vi "PtoP.vi"(3 "Spacing":dbl, 5 "LineNo":i32, 6 "Direction":enum16{"Y to X", "X to Y"}(ring), 7 "Step":dbl, 8 "error in":errorcluster, 9 "Wait time":i32, 10 "Length":i32, 11 "StartPos":dbl[](array[numeric])) -> (0 "error out":errorcluster)   [LabVIEW 2022 SP3]
uses:
  Global 3.vi
  Newport.XPS.CommandInterface
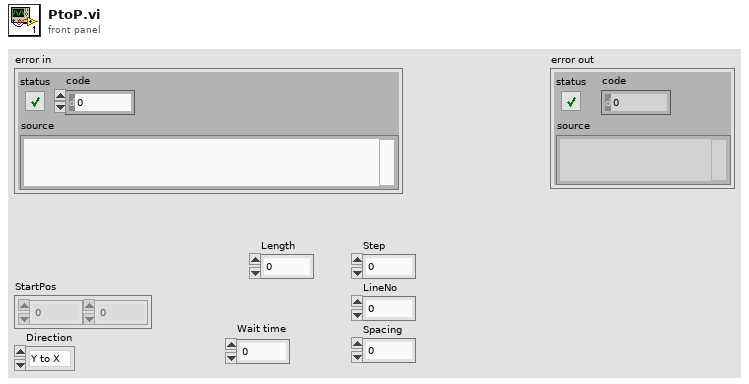
[diagram p1: front panel]
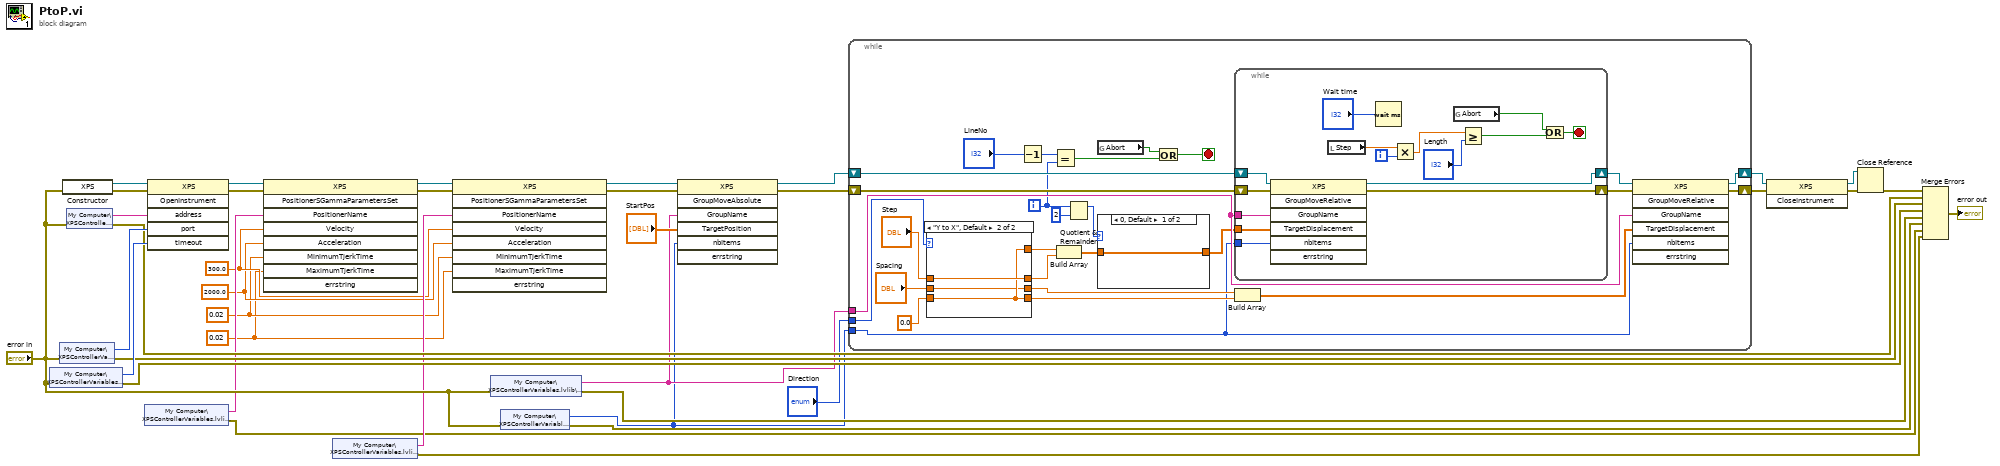
[diagram p0: block diagram]
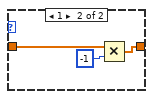
[diagram p2: hidden frame]
diagram:
  w11 = 0.02 ("MaxJT")
  w12 = 0.02 ("MinJT")
  w13 = 2000.0 ("Acc")
  w14 = 300.0 ("Vel")
  n1 = shared-variable "My Computer\\XPSControllerVariables.lvlib\\Timeout"(error in="error in") -> (w33:i16, error out=w28:errorcluster)
  n2 = shared-variable "My Computer\\XPSControllerVariables.lvlib\\Port"(error in="error in") -> (w34:i16, error out=w29:errorcluster)
  n3 = constructor class="XPS"(error in="error in") -> (reference out=w37:refnum<k24>, error out=w36:errorcluster)  [unwired: 2 in, 1 out]
  n4 = shared-variable "My Computer\\XPSControllerVariables.lvlib\\IP"(error in="error in") -> (w35:string, error out=w30:errorcluster)
  n5 = shared-variable "My Computer\\XPSControllerVariables.lvlib\\PosNameX"() -> (w16:string, error out=w9:errorcluster)  [unwired: 1 in]
  n6 = invoke class="XPS" method="OpenInstrument"(reference=w37, error in=w36, "address"=w35, "port"=w34, "timeout"=w33) -> (reference out=w22:refnum<k24>, error out=w21:errorcluster)  [unwired: 1 in, 4 out]
  n7 = invoke class="XPS" method="PositionerSGammaParametersSet"(reference=w22, error in=w21, "PositionerName"=w16, "Velocity"=w14, "Acceleration"=w13, "MinimumTjerkTime"=w12, "MaximumTjerkTime"=w11) -> (reference out=w20:refnum<k24>, error out=w19:errorcluster)  [unwired: 2 in, 7 out]
  n8 = shared-variable "My Computer\\XPSControllerVariables.lvlib\\PosNameY"() -> (w15:string, error out=w8:errorcluster)  [unwired: 1 in]
  n9 = invoke class="XPS" method="PositionerSGammaParametersSet"(reference=w20, error in=w19, "PositionerName"=w15, "Velocity"=w14, "Acceleration"=w13, "MinimumTjerkTime"=w12, "MaximumTjerkTime"=w11) -> (reference out=w18:refnum<k24>, error out=w17:errorcluster)  [unwired: 2 in, 7 out]
  n10 = shared-variable "My Computer\\XPSControllerVariables.lvlib\\GroupName"(error in="error in") -> (w3:string, error out=w27:errorcluster)
  n11 = shared-variable "My Computer\\XPSControllerVariables.lvlib\\nbitem"(error in="error in") -> (w2:i16, error out=w23:errorcluster)
  n12 = invoke class="XPS" method="GroupMoveAbsolute"(reference=w18, error in=w17, "GroupName"=w3, "TargetPosition"="StartPos", "nbItems"=w2) -> (reference out=w7:refnum<k24>, error out=w6:errorcluster)  [unwired: 2 in, 5 out]
  n13 = while {
    tunnel: w3 -> [w45]
    tunnel: w2 -> [w39]
    shift-right: [w47] -> w5
    shift-left: w7 -> [w64]
    shift-right: [w46] -> w4
    shift-left: w6 -> [w63]
    tunnel: "Direction" -> [w49]
    i -> [w44]
    stop <- w57 stop-if-true
    n14 = case shown="\"Y to X\", Default" w49 {
      tunnel: [w86 w88] -> w56
      tunnel: "Step" -> [w86 w89]
      tunnel: [w85 w89] -> w54
      tunnel: 0.0 -> [w85 w88]
      tunnel: [w85 w87] -> w52
      tunnel: [w84 w88] -> w51
      tunnel: "Spacing" -> [w84 w87]
      frame "X to Y" {
      }
      frame "Y to X", Default {
      }
    }
    n15 = Decrement(x="LineNo") -> (x-1=w60:i32)
    n16 = Equal?(x=w60, y=w44) -> (x = y?=w58:bool)
    n17 = Build Array(w56, w54) -> (w42:dbl[])
    n18 = Quotient & Remainder(x=w44, y=2) -> (x-y*floor(x/y)=w40:i32)  [unwired: 1 out]
    n19 = global read "Global 3.vi" "Abort"() -> (w59:bool)
    n20 = case shown="0, Default" w40 {
      tunnel: w42 -> [w80 w82]
      tunnel: [w80 w81] -> w41
      frame 0, Default {
      }
      frame 1 {
        n21 = Multiply(x=w82, y=-1) -> (x*y=w81:dbl[])
      }
    }
    n22 = Or(x=w59, y=w58) -> (x .or. y?=w57:bool)
    n23 = while {
      tunnel: w45 -> [w75]
      tunnel: w41 -> [w74]
      tunnel: w39 -> [w73]
      shift-right: [w77] -> w62
      shift-left: w64 -> [w79]
      shift-right: [w76] -> w61
      shift-left: w63 -> [w78]
      i -> [w71]
      stop <- w65 stop-if-true
      n24 = invoke class="XPS" method="GroupMoveRelative"(reference=w79, error in=w78, "GroupName"=w75, "TargetDisplacement"=w74, "nbItems"=w73) -> (reference out=w77:refnum<k24>, error out=w76:errorcluster)  [unwired: 2 in, 5 out]
      n25 = local read "Step"() -> (w72:dbl)
      n26 = Wait (ms)(milliseconds to wait="Wait time") -> ()  [unwired: 1 out]
      n27 = Multiply(x=w72, y=w71) -> (x*y=w70:dbl)
      n28 = global read "Global 3.vi" "Abort"() -> (w67:bool)
      n29 = Greater Or Equal?(x=w70, y="Length") -> (x >= y?=w66:bool)
      n30 = Or(x=w67, y=w66) -> (x .or. y?=w65:bool)
    }
    n31 = Build Array(w52, w51) -> (w48:dbl[])
    n32 = invoke class="XPS" method="GroupMoveRelative"(reference=w62, error in=w61, "GroupName"=w45, "TargetDisplacement"=w48, "nbItems"=w39) -> (reference out=w47:refnum<k24>, error out=w46:errorcluster)  [unwired: 2 in, 5 out]
  }
  n33 = invoke class="XPS" method="CloseInstrument"(reference=w5, error in=w4) -> (reference out=w32:refnum<k24>, error out=w31:errorcluster)  [unwired: 1 in, 1 out]
  n34 = Close Reference(reference=w32, error in (no error)=w31) -> (error out=w26:errorcluster)
  n35 = Merge Errors(w26, w30, w29, w28, w27, w23, w9, w8) -> (→"error out":errorcluster)
